vi "Get Coeffs.vi"(8 "error in (no error)":errorcluster, 11 "references":T1) -> (0 "error out":errorcluster, 2 "Coefficients":dbl[](array[numeric]), 3 "references out":T1)   [LabVIEW 2013, in "Polynomial Scale editor node.lvclass"]
uses:
  Polynomial Scale editor node.lvclass
  <vilib>/NI/DCAF Table API/Table Manager/object ref.ctl
  <vilib>/NI/Tag Bus Data Framework/Configuration Editor/Classes/Engine Parent/Engine Parent Editor Node.lvclass
  <vilib>/NI/Tag Bus Data Framework/Configuration Editor/Classes/Module editor node/module editor node.lvclass
  module/configuration/Polynomial Scale configuration.lvclass
  <vilib>/NI/DCAF Modules/DCAF Scaling/editor node/Scaling editor node.lvclass
  <vilib>/NI/DCAF Table API/Table Manager/Table Manager.lvclass
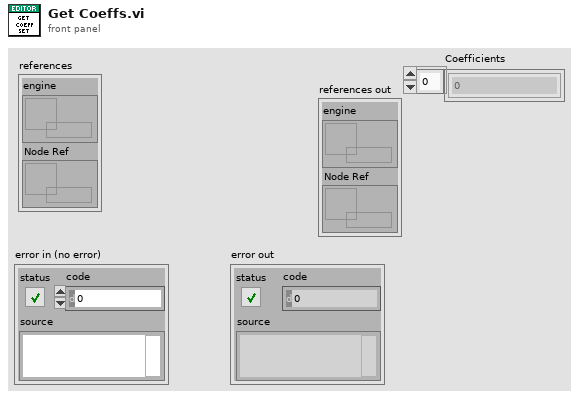
[diagram p1: front panel]
types:
  T1 = typedef "Table Manager.lvlib/Table Manager.lvclass/object ref.ctl" = cluster{"engine":refnum<data-value>, "Node Ref":refnum<data-value>}
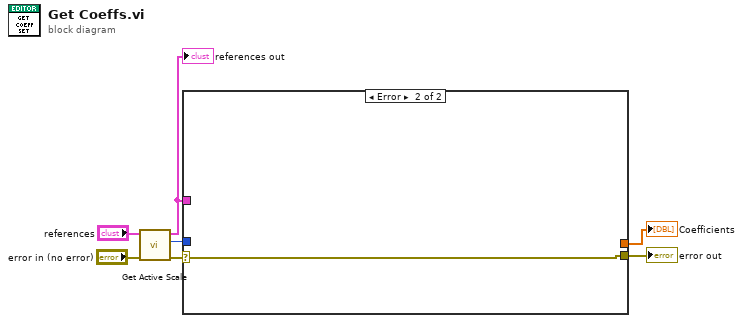
[diagram p0: block diagram]
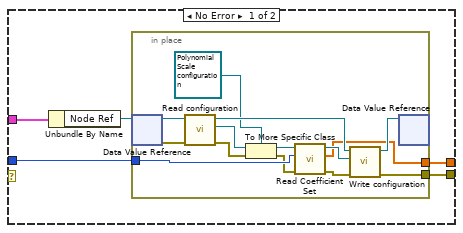
[diagram p2: hidden frame]
diagram:
  n1 = call <vilib>:"Get Active Scale.vi"("error in (no error)"="error in (no error)", "references"="references") -> ("error out"=w3:errorcluster, "Index"=w2:i32, "references out"=w4:T1)  [unwired: 6 in]
  "references out" <- w4
  n2 = case shown="Error" w3 {
    selector: w3 -> [_ w27]
    tunnel: [w12 w27] -> w7
    tunnel: w4 -> [w10 _]
    tunnel: w2 -> [w9 _]
    tunnel: [w8 _] -> w1
    frame No Error {
      n3 = Unbundle By Name(w10) -> ("Node Ref"=w11:refnum<data-value>)
      n4 = in-place {
        in-place-border: [w23] -> w12
        in-place-border: w9 -> [w17]
        in-place-border: [w13] -> w8
        n5 = in-place-dvr #1(w11) -> (w22:refnum<class "module editor node.lvclass">, w26:errorcluster)
        n6 = call-dynamic "Read configuration.vi"("error in"=w26, "NISE_CEF_serializable node in"=w22) -> ("error out"=w24:errorcluster, "configuration"=w25:refnum<class "NISE_CEF_serializable configuration.lvclass">, "NISE_CEF_serializable node out"=w21:refnum<class "module editor node.lvclass">)  [unwired: 7 in]
        n7 = To More Specific Class(target class=refnum<class "Polynomial Scale configuration.lvclass"> refnum ("Polynomial Scale configuration"), reference=w25, error in=w24) -> (specific class reference=w18:refnum<class "Polynomial Scale configuration.lvclass">, error out=w16:errorcluster)
        n8 = call "Read Coefficient Set.vi"("error in (no error)"=w16, "scale index"=w17, "Polynomial Scale configuration in"=w18) -> ("error out"=w15:errorcluster, "Coefficients"=w13:dbl[], "Polynomial Scale configuration out"=w14:refnum<class "Polynomial Scale configuration.lvclass">)  [unwired: 6 in]
        n9 = call-dynamic "Write configuration.vi"("error in"=w15, "configuration"=w14, "NISE_CEF_serializable node in"=w21) -> ("error out"=w23:errorcluster, "NISE_CEF_serializable node out"=w20:refnum<class "module editor node.lvclass">)  [unwired: 7 in]
        n10 = in-place-dvr #1(w20) -> ()  [unwired: 2 out]
      }
    }
    frame Error {
    }
  }
  "error out" <- w7
  "Coefficients" <- w1
